vi "Cowl_Test.vi"(11 "Joystick_IN":T1={"Pilot Left Joystick X"=0.07086614173228346, "Pilot Left Joystick Y"=-0.015748031496062992, "Pilot A Button"=FALSE, "Pilot B Button"=FALSE, "Pilot X Button"=FALSE, "Pilot Y Button"=FALSE, "Pilot Left Bumper"=FALSE, "Pilot Right Bumper"=FALSE, "Pilot View Button"=FALSE, "Pilot Menu Button"=FALSE, "Pilot Left Joystick Press"=FALSE, "Pilot Right Joystick Press"=FALSE, "Pilot Left Trigger"=0.0, "Pilot Right Joystick X"=-0.03937007874015748, "Pilot Right Joystick Y"=0.031496062992125984, "Pilot Right Trigger"=0.0, "Copilot Left Joystick X"=0.047244094488188976, "Copilot Left Joystick Y"=0.10236220472440945, "Copilot A Button"=FALSE, "Copilot B Button"=FALSE, "Copilot X Button"=FALSE, "Copilot Y Button"=FALSE, "Copilot Left Bumper"=FALSE, "Copilot Right Bumper"=FALSE, "Copilot View Button"=FALSE, "Copilot Menu Button"=FALSE, "Copilot Left Joystick Press"=FALSE, "Copilot Right Joystick Press"=FALSE, "Copilot Left Trigger"=0.0, "Copilot Right Joystick X"=-0.007874015748031496, "Copilot Right Joystick Y"=0.047244094488188976, "Copilot Right Trigger"=0.0, "Pilot D-pad North"=FALSE, "Pilot D-pad South"=FALSE, "Pilot D-pad East"=FALSE, "Pilot D-pad West"=FALSE, "Pilot D-pad NE "=FALSE, "Pilot D-pad SE"=FALSE, "Pilot D-pad SW"=FALSE, "Pilot D-pad NW"=FALSE, "CoPilot D-pad North"=FALSE, "CoPilot D-pad South"=FALSE, "CoPilot D-pad East"=FALSE, "CoPilot D-pad West"=FALSE, "CoPilot D-pad NE"=FALSE, "CoPilot D-pad SE"=FALSE, "CoPilot D-pad SW"=FALSE, "CoPilot D-pad NW"=FALSE, "Pilot Left Trigger Pressed"=FALSE, "Pilot Right Trigger Pressed"=FALSE, "CoPilot Left Trigger Pressed"=FALSE, "CoPilot Right Trigger Pressed"=FALSE}) -> ()   [LabVIEW 2019]
uses:
  Cowl_States.ctl
  Cowl_Cluster.ctl
  Cowl_Globals.vi
  Utility VIs/Joystick_Controls.ctl
panel:
  in  "Manual_Power_Down":dbl=0.3
  in  "Manual_Power_Up":dbl=0.395
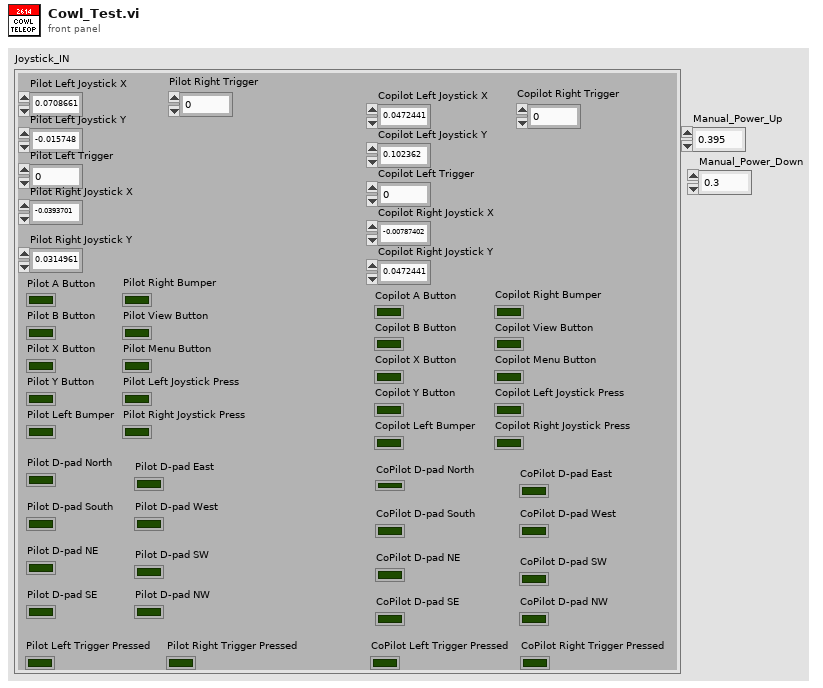
[diagram p1: front panel]
types:
  T1 = typedef "Joystick_Controls.ctl" = cluster{"Pilot Left Joystick X":dbl, "Pilot Left Joystick Y":dbl, "Pilot A Button":bool, "Pilot B Button":bool, "Pilot X Button":bool, "Pilot Y Button":bool, "Pilot Left Bumper":bool, "Pilot Right Bumper":bool, "Pilot View Button":bool, "Pilot Menu Button":bool, "Pilot Left Joystick Press":bool, "Pilot Right Joystick Press":bool, "Pilot Left Trigger":dbl, "Pilot Right Joystick X":dbl, "Pilot Right Joystick Y":dbl, "Pilot Right Trigger":dbl, "Copilot Left Joystick X":dbl, "Copilot Left Joystick Y":dbl, "Copilot A Button":bool, "Copilot B Button":bool, "Copilot X Button":bool, "Copilot Y Button":bool, "Copilot Left Bumper":bool, "Copilot Right Bumper":bool, "Copilot View Button":bool, "Copilot Menu Button":bool, "Copilot Left Joystick Press":bool, "Copilot Right Joystick Press":bool, "Copilot Left Trigger":dbl, "Copilot Right Joystick X":dbl, "Copilot Right Joystick Y":dbl, "Copilot Right Trigger":dbl, "Pilot D-pad North":bool, "Pilot D-pad South":bool, "Pilot D-pad East":bool, "Pilot D-pad West":bool, "Pilot D-pad NE ":bool, "Pilot D-pad SE":bool, "Pilot D-pad SW":bool, "Pilot D-pad NW":bool, "CoPilot D-pad North":bool, "CoPilot D-pad South":bool, "CoPilot D-pad East":bool, "CoPilot D-pad West":bool, "CoPilot D-pad NE":bool, "CoPilot D-pad SE":bool, "CoPilot D-pad SW":bool, "CoPilot D-pad NW":bool, "Pilot Left Trigger Pressed":bool, "Pilot Right Trigger Pressed":bool, "CoPilot Left Trigger Pressed":bool, "CoPilot Right Trigger Pressed":bool}
  T2 = typedef "Cowl_Cluster.ctl" = cluster{"Control_State\n":T3, "Manual_Cowl_%Power":dbl}
  T3 = typedef "Cowl_States.ctl" = enum16{"Manual_%VBus", "GoToAngle"}
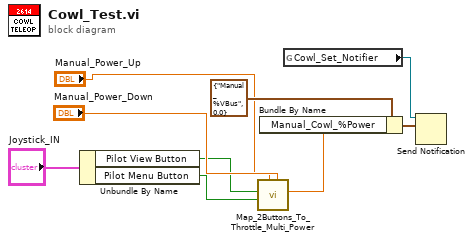
[diagram p0: block diagram]
diagram:
  n1 = Unbundle By Name("Joystick_IN") -> ("Pilot View Button"=w3:bool, "Pilot Menu Button"=w2:bool)
  n2 = call "Map_2Buttons_To_Throttle_Multi_Power.vi"("Power_Down"="Manual_Power_Down", "Power_Up"="Manual_Power_Up", "Down"=w2, "Up"=w3) -> ("Throttle"=w1:dbl)  [unwired: 7 in]
  n3 = Bundle By Name(cluster=T2 {"Control_State\n"=enum."Manual_%VBus", "Manual_Cowl_%Power"=0.0} ("Cluster"), "Manual_Cowl_%Power"=w1) -> (w8:T2)
  n4 = global read "Cowl_Globals.vi" "Cowl_Set_Notifier"() -> (w6:refnum<notifier>)
  n5 = Send Notification(notification=w8, notifier=w6) -> ()  [unwired: 1 in, 2 out]
